vi "Configure Serial Bus (LIN - Trigger - Symbolic).vi"(0 "VISA resource name":refnum<visa-resource-name>, 1 "Value to Trigger (1)":dbl=1.0, 5 "Serial Bus Name (1: Serial Bus 1)":i32(ring)=1 items=["Serial Bus 1"=1, "Serial Bus 2"=2], 7 "Message to Trigger ()":string, 9 "Signal to Trigger ()":string, 11 "error in (no error)":errorcluster) -> (4 "VISA resource name out":refnum<visa-resource-name>, 15 "error out":errorcluster)   [LabVIEW 2015, in "Agilent 2000 3000 X-Series.lvlib"]
doc: "Configures the symbolic trigger settings of LIN bus. Used when the trigger condition is Frame, or \"Frame and Signal\"\n\n<b>Note:</b>\nBefore this VI is called LIN symbolic data (a .ldf file) must be loaded into the oscilloscope using <b>Recall Data From File</b>.vi. A serial bus must be configured for LIN-Symbolic decode before calling this VI.\nThis VI is not supported by 1000 Series models"
uses:
  Agilent 2000 3000 X-Series.lvlib
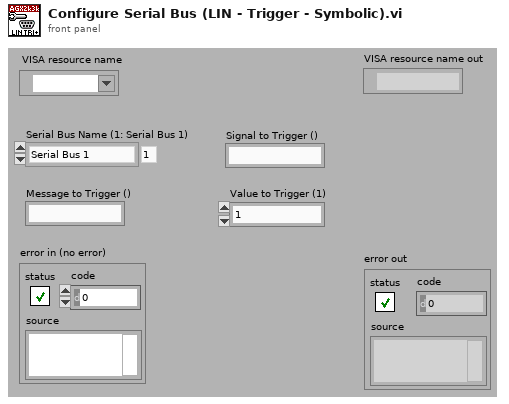
[diagram p1: front panel]
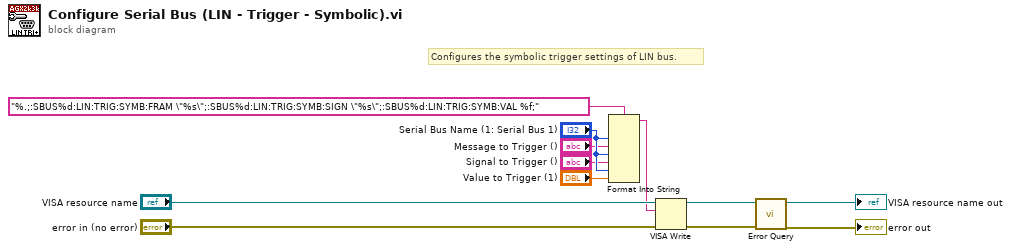
[diagram p0: block diagram]
diagram:
  # "Configures the symbolic trigger settings of LIN bus."
  n1 = Format Into String(format string="%.;:SBUS%d:LIN:TRIG:SYMB:FRAM \"%s\";:SBUS%d:LIN:TRIG:SYMB:SIGN \"%s\";:SBUS%d:LIN:TRIG:SYMB:VAL %f;", "Serial Bus Name (1: Serial Bus 1)", "Message to Trigger ()", "Serial Bus Name (1: Serial Bus 1)", "Signal to Trigger ()", "Serial Bus Name (1: Serial Bus 1)", "Value to Trigger (1)") -> (resulting string=w1:string)  [unwired: 2 in, 1 out]
  n2 = VISA Write(VISA resource name="VISA resource name", write buffer=w1, error in (no error)="error in (no error)") -> (VISA resource name out=w10:refnum<visa-resource-name>, error out=w9:errorcluster)  [unwired: 1 out]
  n3 = call "Error Query.vi"("error in (no error)"=w9, "VISA resource name"=w10) -> ("error out"=→"error out":errorcluster, "VISA resource name out"=→"VISA resource name out":refnum<visa-resource-name>)  [unwired: 8 out]
